vi "Save hit rate.vi"(2 "Data cluster":T3, 3 "Elements to average":i32) -> (1 "data":T1(array[cluster]))   [LabVIEW 2016]
uses:
  Typedefs/Hit chart cluster refnum.ctl
  <vilib>/Analysis/baseanly.llb/Mean (DBL).vi
  Global Variables/Scintillator IDs.vi
  <vilib>/Analysis/NI_AALBase.lvlib
panel:
  in  "error in":errorcluster
  out "error out":errorcluster
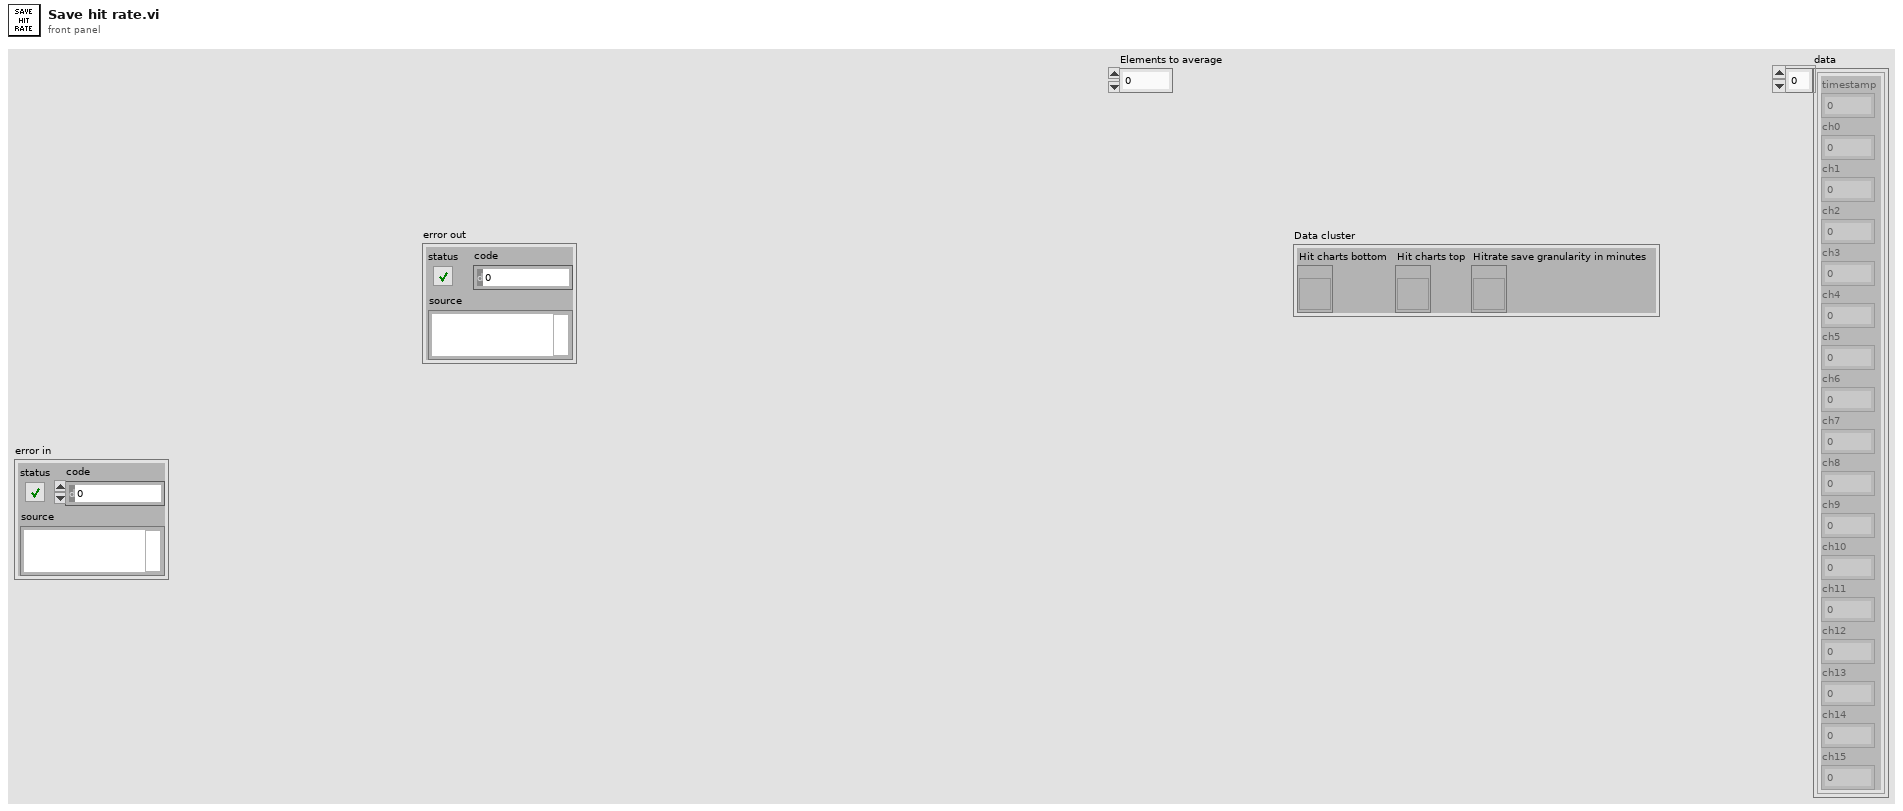
[diagram p1: front panel]
types:
  T1 = cluster{"timestamp":u32, "ch0":dbl, "ch1":dbl, "ch2":dbl, "ch3":dbl, "ch4":dbl, "ch5":dbl, "ch6":dbl, "ch7":dbl, "ch8":dbl, "ch9":dbl, "ch10":dbl, "ch11":dbl, "ch12":dbl, "ch13":dbl, "ch14":dbl, "ch15":dbl}[]
  T2 = typedef "Hit chart cluster refnum.ctl" = refnum<vi>
  T3 = cluster{"Hit charts bottom":T2, "Hit charts top":T2, "Hitrate save granularity in minutes":refnum<vi>}
  T4 = cluster{"timestamp":u32, "ch0":dbl, "ch1":dbl, "ch2":dbl, "ch3":dbl, "ch4":dbl, "ch5":dbl, "ch6":dbl, "ch7":dbl, "ch8":dbl, "ch9":dbl, "ch10":dbl, "ch11":dbl, "ch12":dbl, "ch13":dbl, "ch14":dbl, "ch15":dbl}
  T5 = enum16{"insertPPS", "insertUTC", "read", "initiate"}
  T6 = typedef "HitChart refnum.ctl" = refnum<vi>
  T7 = cluster{"Coincidences":dbl, "Non-coincidences":dbl, "Ratio":dbl, "Total hits":dbl}[]
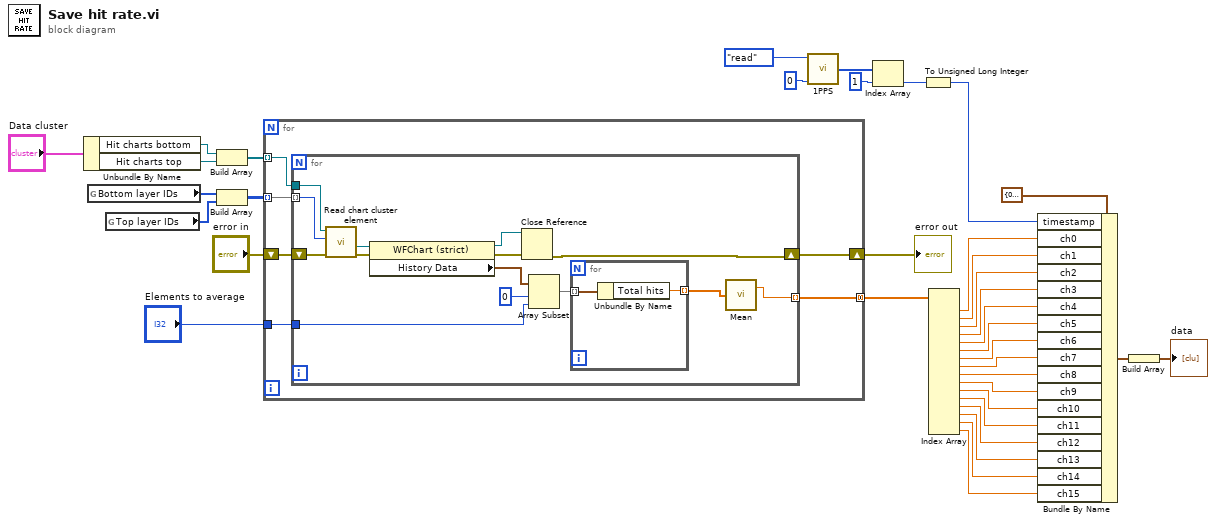
[diagram p0: block diagram]
diagram:
  n1 = Unbundle By Name("Data cluster") -> ("Hit charts bottom"=w23:T2, "Hit charts top"=w22:T2)
  n2 = global read "Scintillator IDs.vi" "Bottom layer IDs"() -> (w27:i8[])
  n3 = global read "Scintillator IDs.vi" "Top layer IDs"() -> (w26:i8[])
  n4 = Build Array(w23, w22) -> (w29:T2[])
  n5 = Build Array(w27, w26) -> (w28:i8[][])
  n6 = for {
    tunnel: w28 -> [w39] mode=indexing
    shift-right: [w41] -> w35
    shift-left: "error in" -> [w42]
    tunnel: w29 -> [w40] mode=indexing
    tunnel: "Elements to average" -> [w38]
    tunnel: [w37] -> w20 mode=concatenating
    n7 = for {
      tunnel: w39 -> [w54] mode=indexing
      shift-right: [w43] -> w41
      shift-left: w42 -> [w55]
      tunnel: w40 -> [w56]
      tunnel: w38 -> [w52]
      tunnel: [w49] -> w37 mode=indexing
      n8 = call "Read chart cluster element.vi"("error in (no error)"=w55, "Channel"=w54, "Chart cluster"=w56) -> ("error out"=w47:errorcluster, "Chart ref"=w48:T6)  [unwired: 5 in, 2 out]
      n9 = property class="WFChart (strict)"(reference=w48, error in=w47) -> (reference out=w44:T6, error out=w45:errorcluster, "History Data"=w46:T7)
      n10 = Close Reference(reference=w44, error in (no error)=w45) -> (error out=w43:errorcluster)
      n11 = Array Subset(array=w46, index=0, length=w52) -> (w51:T7)
      n12 = for {
        tunnel: w51 -> [w58] mode=indexing
        tunnel: [w57] -> w50 mode=indexing
        n13 = Unbundle By Name(w58) -> ("Total hits"=w57:dbl)
      }
      n14 = call-poly <vilib>:"Mean.vi"("X"=w50) -> ("mean"=w49:dbl)  [unwired: 1 out]
    }
  }
  "error out" <- w35
  n15 = call "1PPS.vi"("Read Index\nNumber"=0 ("Read Index\nNumber"), "Action"=T5."read") -> ("Array"=w32:u32[])  [unwired: 2 in]
  n16 = Index Array(array=w32, index=1) -> (element=w30:u32)
  n17 = To Unsigned Long Integer(number=w30) -> (unsigned 32bit integer=w19:u32)
  n18 = Index Array(array=w20) -> (element #1=w18:dbl, element #2=w17:dbl, element #3=w16:dbl, element #4=w15:dbl, element #5=w14:dbl, element #6=w13:dbl, element #7=w12:dbl, element #8=w11:dbl, element #9=w10:dbl, element #10=w9:dbl, element #11=w8:dbl, element #12=w7:dbl, element #13=w6:dbl, element #14=w5:dbl, element #15=w4:dbl, element #16=w3:dbl)  [unwired: 16 in]
  n19 = Bundle By Name(cluster=T4 {"timestamp"=0, "ch0"=0.0, "ch1"=0.0, "ch2"=0.0, "ch3"=0.0, "ch4"=0.0, "ch5"=0.0, "ch6"=0.0, "ch7"=0.0, "ch8"=0.0, "ch9"=0.0, "ch10"=0.0, "ch11"=0.0, "ch12"=0.0, "ch13"=0.0, "ch14"=0.0, "ch15"=0.0}, "timestamp"=w19, "ch0"=w18, "ch1"=w17, "ch2"=w16, "ch3"=w15, "ch4"=w14, "ch5"=w13, "ch6"=w12, "ch7"=w11, "ch8"=w10, "ch9"=w9, "ch10"=w8, "ch11"=w7, "ch12"=w6, "ch13"=w5, "ch14"=w4, "ch15"=w3) -> (w2:T4)
  n20 = Build Array(w2) -> (→"data":T1)
